vi "UnitTest-BackupOnLaunch.vi"(8 "error in (no error)":errorcluster) -> (0 "error out":errorcluster)   [LabVIEW 2014]
uses:
  TableLogger_Actor/TableLoggerConfig.ctl
  TableLogger_Actor/TableLoggerTypes.ctl
  TableLogger_Actor/TableLoggerBackupConfig.ctl
  <vilib>/addons/_JKI Toolkits/Caraya/classes/Test/Test.lvclass
  TableLogger_Actor/TableLogger_Actor.lvlib
panel:
  # "Connector Pane"
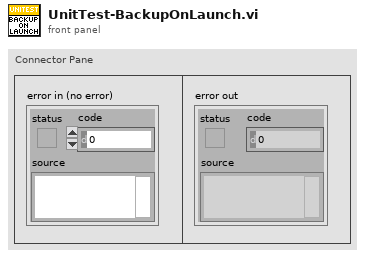
[diagram p1: front panel]
types:
  T1 = typedef "TableLogger_Actor.lvlib/TableLoggerConfig.ctl" = cluster{"TableLogger":T2, "DB File Path":path, "DB Backup Config":T3}
  T2 = typedef "TableLogger_Actor.lvlib/TableLoggerTypes.ctl" = enum16{"CSV Logger", "SQLite Logger"}
  T3 = typedef "TableLogger_Actor.lvlib/TableLoggerBackupConfig.ctl" = cluster{"Directory":path, "UTC Time Format":bool, "On Launch":bool, "Interval (Hours)":dbl, "Size Multiples (Bytes)":i32}
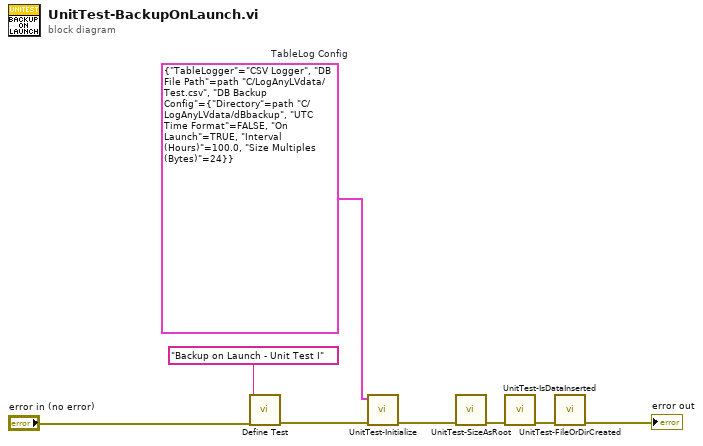
[diagram p0: block diagram]
diagram:
  w4 = T1 {"TableLogger"=enum."CSV Logger", "DB File Path"=path "C:/LogAnyLVdata/Test.csv", "DB Backup Config"={"Directory"=path "C:/LogAnyLVdata/dBbackup", "UTC Time Format"=FALSE, "On Launch"=TRUE, "Interval (Hours)"=100.0, "Size Multiples (Bytes)"=24}}  # TableLog Config
  n1 = call <vilib>:"Define Test.vi"("error in (no error)"="error in (no error)", "Label (VI Title)"="Backup on Launch - Unit Test I") -> ("error out"=w5:errorcluster)  [unwired: 9 in]
  n2 = call "UnitTest-Initialize.vi"("error in"=w5, "Config IN"=w4) -> ("error out"=w3:errorcluster)  [unwired: 7 in, 2 out]
  n3 = call "UnitTest-SizeAsRoot.vi"("error in"=w3) -> ("error out"=w2:errorcluster)  [unwired: 10 in]
  n4 = call "UnitTest-IsDataInserted.vi"("error in"=w2) -> ("error out"=w1:errorcluster)  [unwired: 10 in]
  n5 = call "UnitTest-FileOrDirCreated.vi"("error in"=w1) -> ("error out"=→"error out":errorcluster)  [unwired: 10 in]
